vi "Configure Decision Feedback Equalization.vi"(0 "VISA resource name":refnum<visa-resource-name>, 1 "Gain (0.0)":dbl, 5 "Enable DFE (T: Enable)":bool=TRUE, 7 "DFE Source (1: Channel 1)":i32(ring)=1 items=["Channel 1"=1, "Channel 2"=2, "Channel 3"=3, "Channel 4"=4, "Function 1"=5, "Function 2"=6, "Function 3"=7, "Function 4"=8, "Memory 1"=9, "Memory 2"=10, "Memory 3"=11, "Memory 4"=12, "Differential 1"=13, "Differential 2"=14, "Common 1"=15, "Common 2"=16], 9 "Drift (1 ms)":dbl=0.001, 11 "error in (no error)":errorcluster, 12 "Lower Target (-1.0)":dbl=-1.0, 13 "Upper Target (1.0)":dbl=1.0) -> (4 "VISA resource name out":refnum<visa-resource-name>, 15 "error out":errorcluster)   [LabVIEW 2020, in "Agilent 90000 Series.lvlib"]
doc: "Configures the basic settings for Feed-Forward Equalization."
uses:
  Agilent 90000 Series.lvlib
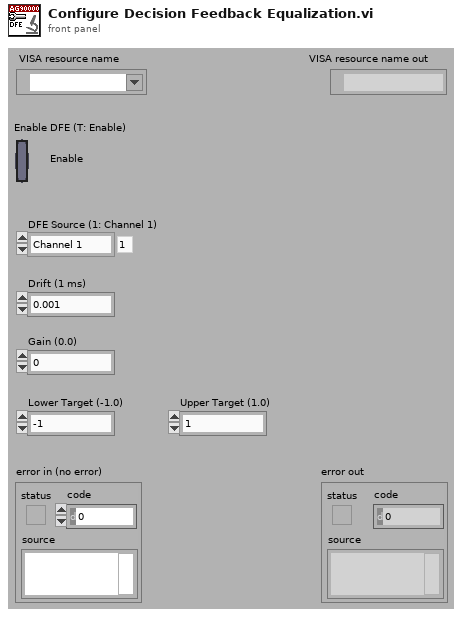
[diagram p1: front panel]
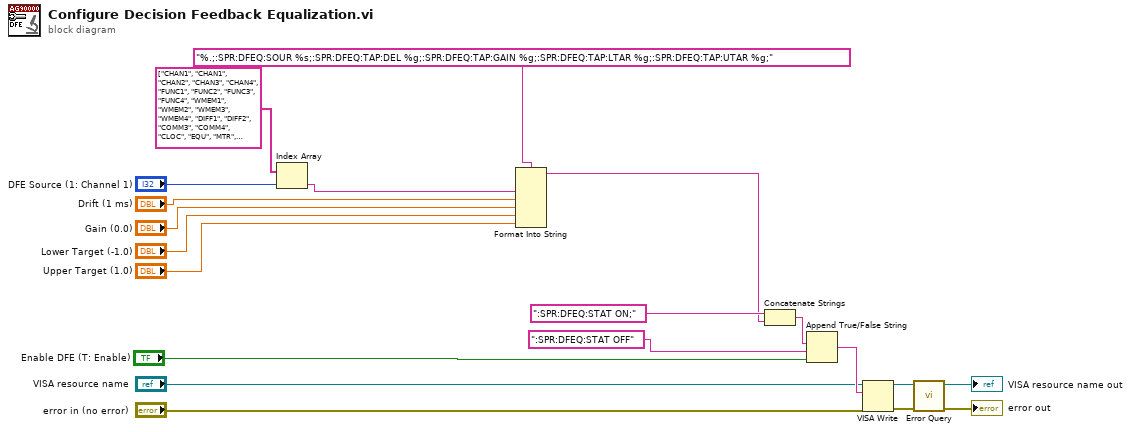
[diagram p0: block diagram]
diagram:
  n1 = Index Array(array=string[] ["CHAN1", "CHAN1", "CHAN2", "CHAN3", "CHAN4", "FUNC1", "FUNC2", "FUNC3", "FUNC4", "WMEM1", "WMEM2", "WMEM3", "WMEM4", "DIFF1", "DIFF2", "COMM3", "COMM4", "CLOC", "EQU", "MTR", "MSP"] ("subarray 2"), index="DFE Source (1: Channel 1)") -> (element=w5:string)
  n2 = Format Into String(format string="%.;:SPR:DFEQ:SOUR %s;:SPR:DFEQ:TAP:DEL %g;:SPR:DFEQ:TAP:GAIN %g;:SPR:DFEQ:TAP:LTAR %g;:SPR:DFEQ:TAP:UTAR %g;", w5, "Drift (1 ms)", "Gain (0.0)", "Lower Target (-1.0)", "Upper Target (1.0)") -> (resulting string=w6:string)  [unwired: 2 in, 1 out]
  n3 = Concatenate Strings(":SPR:DFEQ:STAT ON;" ("false string"), w6) -> (w11:string)
  n4 = Append True/False String(1:"Enable DFE (T: Enable)", 2:":SPR:DFEQ:STAT OFF" ("false string"), 3:w11) -> (0:w9:string)  [unwired: 1 out]
  n5 = VISA Write(VISA resource name="VISA resource name", write buffer=w9, error in (no error)="error in (no error)") -> (VISA resource name out=w18:refnum<visa-resource-name>, error out=w17:errorcluster)  [unwired: 1 out]
  n6 = call "Error Query.vi"("error in (no error)"=w17, "VISA resource name"=w18) -> ("error out"=→"error out":errorcluster, "VISA resource name out"=→"VISA resource name out":refnum<visa-resource-name>)  [unwired: 8 out]
